vi "Tester.vi"() -> ()   [LabVIEW 2020, in "Thermal Chamber Response Simlator.lvclass"]
uses:
  Thermal Chamber Response Simlator.lvclass
  Thermal Chamber Response Simlator.lvclass/Thermal Chamber Response Simlator.ctl
  Private/Get Current Time if Not Set.vi
panel:
  out "Waveform Chart":dbl(graph)
  in  "stop":bool
  in  "Ramp Rate [degC/s]":dbl
  in  "Heating?":bool
  in  "Setpoint [degC]":dbl
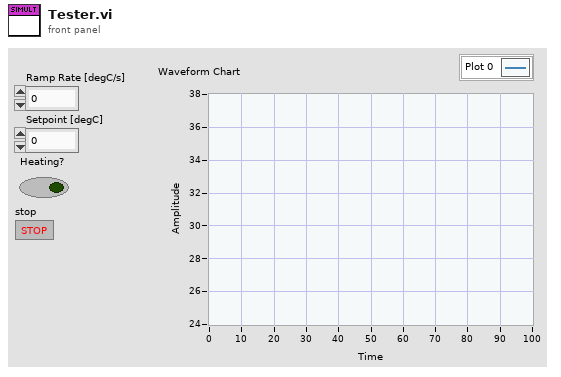
[diagram p1: front panel]
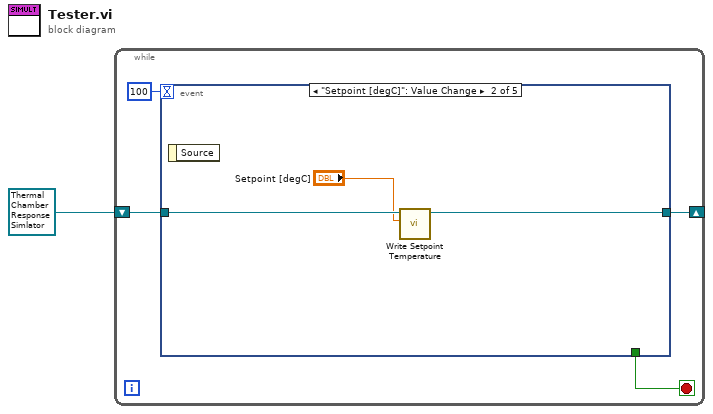
[diagram p0: block diagram]
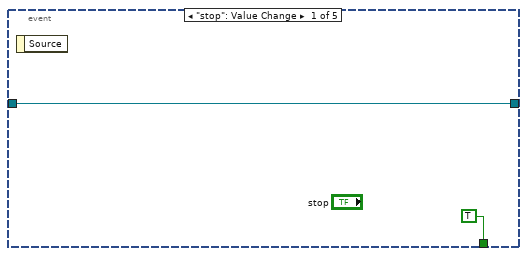
[diagram p2: hidden frame]
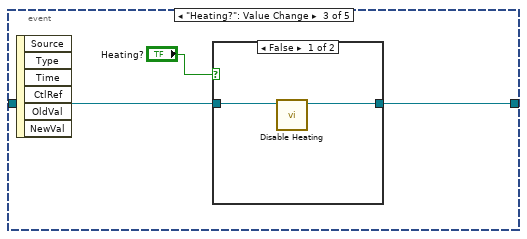
[diagram p3: hidden frame]
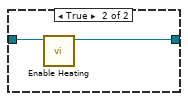
[diagram p4: hidden frame]
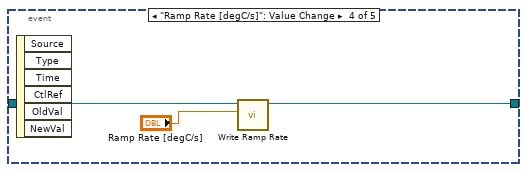
[diagram p5: hidden frame]
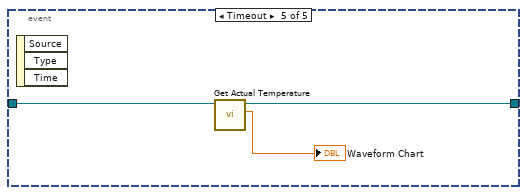
[diagram p6: hidden frame]
diagram:
  n1 = while {
    shift-right: [w3] -> _
    shift-left: refnum<class "Thermal Chamber Response Simlator.lvclass"> refnum ("Thermal Chamber Response Simlator.lvclass") -> [w4]
    stop <- w5 stop-if-true
    n2 = event shown="[1] \"Setpoint [degC]\": Value Change" {
      selector: _ -> [_ _ _ _ _]
      dyn-events: _ -> [_ _ _ _ _]
      timeout: 100 -> [_ _ _ _ _]
      tunnel: [TRUE _ _ _ _] -> w5
      tunnel: w4 -> [w6 w10 w13 w19 w23]
      tunnel: [w6 w9 w12 w20 w22] -> w3
      event "stop": Value Change {
        n3 = event-data() -> ()  [unwired: 1 in, 1 out]
      }
      event "Setpoint [degC]": Value Change {
        n4 = event-data() -> ()  [unwired: 1 in, 1 out]
        n5 = call "Write Setpoint Temperature.vi"("Setpoint Temperature [degC]"="Setpoint [degC]", "Thermal Chamber Response Simlator In"=w10) -> ("Thermal Chamber Response Simlator Out"=w9:refnum<class "Thermal Chamber Response Simlator.lvclass">)  [unwired: 8 in, 1 out]
      }
      event "Heating?": Value Change {
        n6 = event-data() -> ()  [unwired: 1 in, 6 out]
        n7 = case shown="False" "Heating?" {
          tunnel: w13 -> [w15 w17]
          tunnel: [w14 w16] -> w12
          frame False {
            n8 = call "Disable Heating.vi"("Thermal Chamber Response Simlator In"=w15) -> ("Thermal Chamber Response Simlator Out"=w14:refnum<class "Thermal Chamber Response Simlator.lvclass">)  [unwired: 9 in, 1 out]
          }
          frame True {
            n9 = call "Enable Heating.vi"("Thermal Chamber Response Simlator In"=w17) -> ("Thermal Chamber Response Simlator Out"=w16:refnum<class "Thermal Chamber Response Simlator.lvclass">)  [unwired: 9 in, 1 out]
          }
        }
      }
      event "Ramp Rate [degC/s]": Value Change {
        n10 = event-data() -> ()  [unwired: 1 in, 6 out]
        n11 = call "Write Ramp Rate.vi"("Ramp Rate [degC/s]"="Ramp Rate [degC/s]", "Thermal Chamber Response Simlator In"=w19) -> ("Thermal Chamber Response Simlator Out"=w20:refnum<class "Thermal Chamber Response Simlator.lvclass">)  [unwired: 8 in, 1 out]
      }
      event Timeout {
        n12 = event-data() -> ()  [unwired: 1 in, 3 out]
        n13 = call "Get Actual Temperature.vi"("Thermal Chamber Response Simlator In"=w23) -> ("Actual Temperature [degC]"=→"Waveform Chart":dbl, "Thermal Chamber Response Simlator Out"=w22:refnum<class "Thermal Chamber Response Simlator.lvclass">)  [unwired: 8 in, 1 out]
      }
    }
  }
